vi "FaultReset.vi"(8 "error in (no error)":errorcluster, 11 "IgusMotorDrive in":refnum<class "IgusMotorDrive.lvclass">) -> (0 "error out":errorcluster, 3 "IgusMotorDrive out":refnum<class "IgusMotorDrive.lvclass">)   [LabVIEW 2016, in "IgusMotorDrive.lvclass"]
uses:
  IgusMotorDrive.lvclass
  typedefs/Controlword--enum.ctl
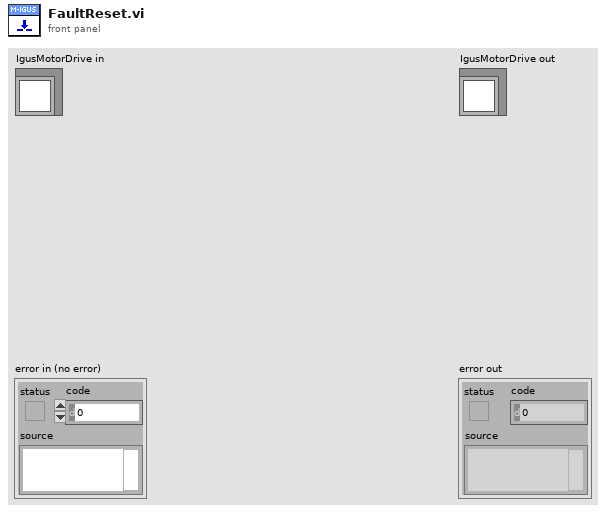
[diagram p1: front panel]
types:
  T1 = typedef "IgusMotorDrive.lvclass/Controlword--enum.ctl" = enum16{"Shutdown", "Switch On", "Switch On and Enable Operation", "Disable Voltage", "Halt", "Quick Stop", "Disable Operation", "Enable Operation", "Fault Reset"}
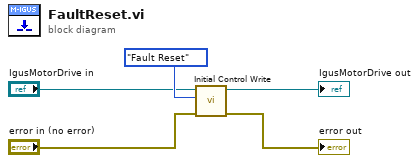
[diagram p0: block diagram]
diagram:
  n1 = call "Initial Control Write.vi"("error in"="error in (no error)", "Controlword"=Controlword--enum."Fault Reset", "IgusMotorDrive in"="IgusMotorDrive in") -> ("error out"=→"error out":errorcluster, "IgusMotorDrive out"=→"IgusMotorDrive out":refnum<class "IgusMotorDrive.lvclass">)  [unwired: 4 in, 3 out]
